vi "Configure Output Sweep.vi"(0 "VISA resource name":refnum<visa-resource-name>, 1 "Source Mode  (0: Voltage)":u16(ring) items=["Voltage", "Current"], 2 "Dual Sweep (F:Disable)":bool, 5 "Number of Points (5)":u32=5, 7 "Start Amplitude (1)":dbl=1.0, 9 "Stop Amplitude (2)":dbl=2.0, 11 "error in (no error)":errorcluster, 12 "Sweep Spacing  (0: Linear)":u16(ring) items=["Linear", "Logarithmic"], 13 "Source Delay (0)":dbl=1.0) -> (4 "VISA resource name out":refnum<visa-resource-name>, 15 "error out":errorcluster)   [LabVIEW 2022 SP3, in "Keithley 2450.lvlib"]
doc: "This VI sets up a linear/logarithmic sweep for a set number of measurement points."
uses:
  Keithley 2450.lvlib
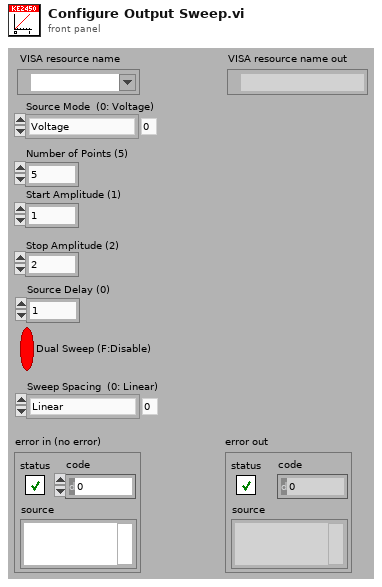
[diagram p1: front panel]
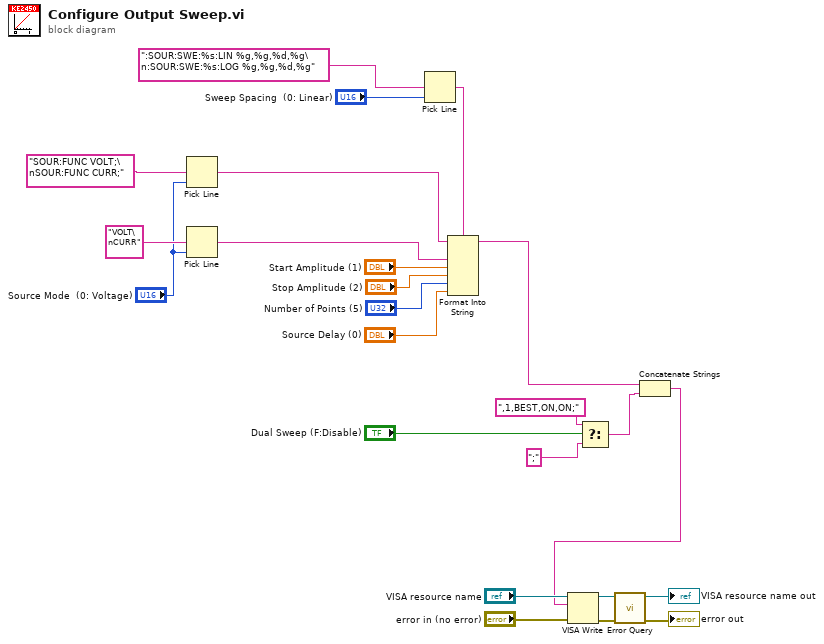
[diagram p0: block diagram]
diagram:
  n1 = Pick Line(multi-line string="SOUR:FUNC VOLT;\nSOUR:FUNC CURR;", line index="Source Mode  (0: Voltage)") -> (output string=w5:string)  [unwired: 1 out]
  n2 = Pick Line(multi-line string="VOLT\nCURR", line index="Source Mode  (0: Voltage)") -> (output string=w13:string)  [unwired: 1 out]
  n3 = Pick Line(multi-line string=":SOUR:SWE:%s:LIN %g,%g,%d,%g\n:SOUR:SWE:%s:LOG %g,%g,%d,%g", line index="Sweep Spacing  (0: Linear)") -> (output string=w14:string)  [unwired: 1 in]
  n4 = Format Into String(format string=w14, initial string=w5, w13, "Start Amplitude (1)", "Stop Amplitude (2)", "Number of Points (5)", "Source Delay (0)") -> (resulting string=w6:string)  [unwired: 1 in, 1 out]
  n5 = Select(t=",1,BEST,ON,ON;", s="Dual Sweep (F:Disable)", f=";") -> (s? t:f=w3:string)
  n6 = Concatenate Strings(w6, w3) -> (w4:string)
  n7 = VISA Write(VISA resource name="VISA resource name", write buffer=w4, error in (no error)="error in (no error)") -> (VISA resource name out=w18:refnum<visa-resource-name>, error out=w17:errorcluster)  [unwired: 1 out]
  n8 = call "Error Query.vi"("error in (no error)"=w17, "VISA resource name"=w18) -> ("error out"=→"error out":errorcluster, "VISA resource name out"=→"VISA resource name out":refnum<visa-resource-name>)  [unwired: 8 out]
